vi "move axe.vi"(9 "Axe":dbl, 10 "Vitesse":dbl, 11 "Angle":dbl) -> ()   [LabVIEW 2016]
uses:
  Settings/Traverse-Settings-Global.vi
  <userlib>/ICNC/ICNC2.lvlib
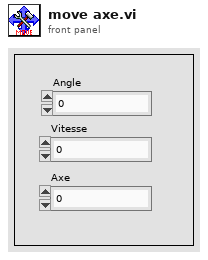
[diagram p1: front panel]
types:
  T1 = cluster{"Acceleration":dbl[], "Deceleration":dbl[], "Max Velocity":dbl[], "Speed":dbl, "Pulse/Degree":dbl, "Degre Factor":dbl[]}
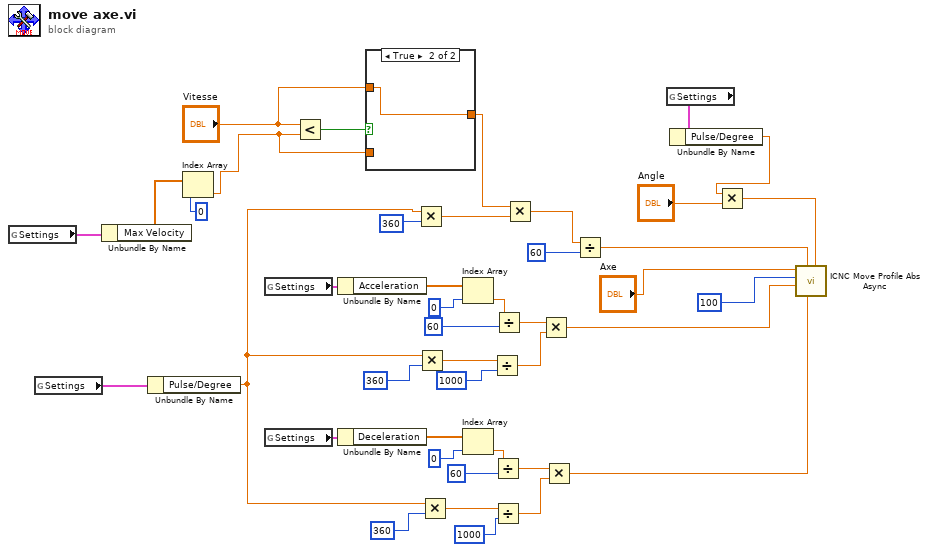
[diagram p0: block diagram]
diagram:
  n1 = global read "Traverse-Settings-Global.vi" "Settings"() -> (w1:T1)
  n2 = global read "Traverse-Settings-Global.vi" "Settings"() -> (w5:T1)
  n3 = Unbundle By Name(w1) -> ("Max Velocity"=w15:dbl[])
  n4 = Unbundle By Name(w5) -> ("Pulse/Degree"=w4:dbl)
  n5 = Index Array(array=w15, index=0) -> (element=w14:dbl)
  n6 = global read "Traverse-Settings-Global.vi" "Settings"() -> (w13:T1)
  n7 = global read "Traverse-Settings-Global.vi" "Settings"() -> (w9:T1)
  n8 = Less?(x="Vitesse", y=w14) -> (x < y?=w28:bool)
  n9 = Unbundle By Name(w13) -> ("Acceleration"=w12:dbl[])
  n10 = Unbundle By Name(w9) -> ("Deceleration"=w8:dbl[])
  n11 = case shown="True" w28 {
    tunnel: "Vitesse" -> [_ w44]
    tunnel: w14 -> [w43 _]
    tunnel: [w43 w44] -> w23
    frame False {
    }
    frame True {
    }
  }
  n12 = Multiply(x=w4, y=360) -> (x*y=w24:dbl)
  n13 = Multiply(x=w4, y=360) -> (x*y=w26:dbl)
  n14 = Multiply(x=w4, y=360) -> (x*y=w25:dbl)
  n15 = Index Array(array=w12, index=0) -> (element=w10:dbl)
  n16 = Index Array(array=w8, index=0) -> (element=w6:dbl)
  n17 = Divide(x=w26, y=1000) -> (x/y=w41:dbl)
  n18 = Divide(x=w6, y=60) -> (x/y=w37:dbl)
  n19 = Divide(x=w25, y=1000) -> (x/y=w36:dbl)
  n20 = Divide(x=w10, y=60) -> (x/y=w31:dbl)
  n21 = Multiply(x=w23, y=w24) -> (x*y=w30:dbl)
  n22 = Multiply(x=w31, y=w41) -> (x*y=w20:dbl)
  n23 = Multiply(x=w37, y=w36) -> (x*y=w19:dbl)
  n24 = Divide(x=w30, y=60) -> (x/y=w22:dbl)
  n25 = global read "Traverse-Settings-Global.vi" "Settings"() -> (w3:T1)
  n26 = Unbundle By Name(w3) -> ("Pulse/Degree"=w2:dbl)
  n27 = Multiply(x=w2, y="Angle") -> (x*y=w17:dbl)
  n28 = call "ICNC Move Profile Abs Async.vi"("Position"=w17, "Decel"=w19, "Speed"=w22, "Accel"=w20, "FStartStop"=100, "Axe"="Axe") -> ()  [unwired: 4 in, 2 out]
